vi "Update Verbose Explanation.vi"(8 "error in (no error)":errorcluster, 9 "Verbose":refnum<class "TestManagerMsg.Verbose.lvclass">, 11 "Test Event Storage in":refnum<class "Test Event Storage.lvclass">) -> (0 "error out":errorcluster, 3 "Test Event Storage out":refnum<class "Test Event Storage.lvclass">)   [LabVIEW 2013, in "Caraya.lvlib" / "Test Event Storage.lvclass"]
uses:
  Test Event Storage.lvclass
  Test Manager Message Verbose/TestManagerMsg.Verbose.lvclass
  Test Event Storage.lvclass/Test Event Storage.ctl
  assert store -- cluster.ctl
  Test Manager Message Assertion/TestManagerMsg.Assertion.lvclass
  Test Manager Message/TestManagerMsg.lvclass/TestManagerMsg.ctl
  Test Manager Message/TestManagerMsg.lvclass
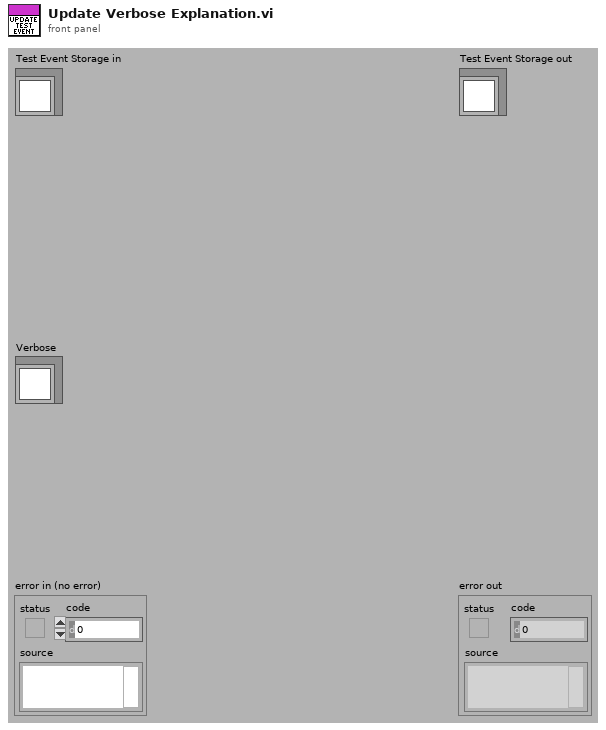
[diagram p1: front panel]
types:
  T1 = typedef "Caraya.lvlib/Test Event Storage.lvclass/assert store -- cluster.ctl" = cluster{"Assertion":refnum<class "TestManagerMsg.Assertion.lvclass">, "Explanation":refnum<class "TestManagerMsg.Verbose.lvclass">, "properties":variant, "measurements":variant, "user-defined":variant}
  T2 = typedef "Caraya.lvlib/Test Event Storage.lvclass/Store Type -- enum.ctl" = enum16{"Suite", "Test", "Assert", "none"}
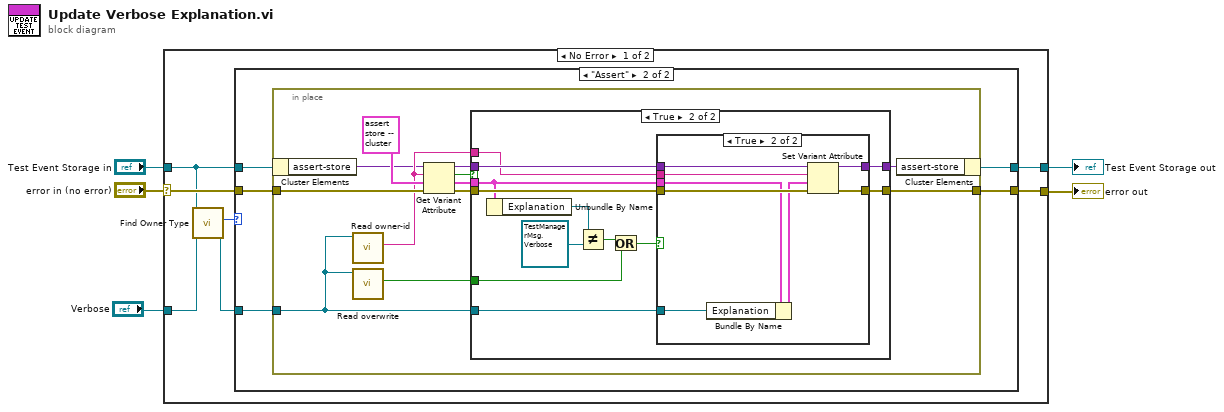
[diagram p0: block diagram]
diagram:
  n1 = case shown="No Error" "error in (no error)" {
    selector: "error in (no error)" -> [w12 w57]
    tunnel: [w11 w57] -> w4
    tunnel: [w10 w56] -> w2
    tunnel: "Test Event Storage in" -> [w9 w56]
    tunnel: "Verbose" -> [w7 _]
    frame No Error {
      n2 = call "Find Owner Type.vi"("Message"=w7, "Test Event Storage in"=w9) -> ("Message dup"=w6:refnum<class "TestManagerMsg.Verbose.lvclass">, "Owner Type"=w8:T2)  [unwired: 7 in, 1 out]
      n3 = case shown="\"Assert\"" w8 {
        tunnel: w6 -> [_ w19]
        tunnel: w12 -> [w13 w18]
        tunnel: [w13 w17] -> w11
        tunnel: [w14 w16] -> w10
        tunnel: w9 -> [w14 w15]
        frame Default {
          # "Explanations only supported for Assertions at the moment."
        }
        frame "Assert" {
          n4 = in-place {
            in-place-border: w18 -> [w29]
            in-place-border: [w30] -> w17
            in-place-border: w19 -> [w28]
            n5 = in-place-cluster #1(w15) -> ("assert-store"=w20:variant)
            n6 = call "Read owner-id.vi"("TestManagerMsg in"=w28) -> ("owner-id"=w21:string)  [unwired: 9 in, 1 out]
            n7 = call "Read overwrite.vi"("TestManagerMsg in"=w28) -> ("overwrite?"=w23:bool)  [unwired: 9 in, 1 out]
            n8 = Get Variant Attribute(Variant=w20, name=w21, default value (empty Variant)=T1 {"Assertion"=refnum, "Explanation"=refnum, "properties"=variant, "measurements"=variant, "user-defined"=variant} ("assert-store"), error in=w29) -> (duplicate Variant=w27:variant, found=w26:bool, value=w25:T1, error out=w24:errorcluster)
            n9 = case shown="True" w26 {
              tunnel: [w33 w45] -> w31
              tunnel: [w32 w44] -> w30
              tunnel: w24 -> [w32 w43]
              tunnel: w27 -> [w33 w42]
              tunnel: w21 -> [_ w41]
              tunnel: w25 -> [_ w40]
              tunnel: w28 -> [_ w39]
              tunnel: w23 -> [_ w35]
              frame False {
              }
              frame True {
                n10 = Unbundle By Name(w40) -> ("Explanation"=w38:refnum<class "TestManagerMsg.Verbose.lvclass">)
                n11 = Not Equal?(x=w38, y=refnum<class "TestManagerMsg.Verbose.lvclass"> refnum ("x")) -> (x != y?=w36:bool)
                n12 = Or(x=w36, y=w35) -> (x .or. y?=w34:bool)
                n13 = case shown="True" w34 {
                  tunnel: [w47 w55] -> w45
                  tunnel: [w46 w54] -> w44
                  tunnel: w43 -> [w46 w53]
                  tunnel: w42 -> [w47 w52]
                  tunnel: w41 -> [_ w51]
                  tunnel: w40 -> [_ w50]
                  tunnel: w39 -> [_ w48]
                  frame False {
                  }
                  frame True {
                    n14 = Bundle By Name(cluster=w50, "Explanation"=w48) -> (w49:T1)
                    n15 = Set Variant Attribute(Variant=w52, name=w51, value=w49, error in=w53) -> (Variant out=w55:variant, error out=w54:errorcluster)  [unwired: 1 out]
                  }
                }
              }
            }
            n16 = in-place-cluster #1("assert-store"=w31) -> (w16:refnum<class "Test Event Storage.lvclass">)
          }
        }
      }
    }
    frame Error {
    }
  }
  "error out" <- w4
  "Test Event Storage out" <- w2
